vi "opc_client_2.vi"(8 "error in (no error)":errorcluster, 10 "server endpoint URL":string) -> (0 "error out":errorcluster, 1 "Debit":dbl, 2 "Courant":dbl, 4 "Tension":dbl, 5 "temperature":dbl, 6 "Pression":dbl, 7 "etat":string, 11 "OPC UA client refnum out":T1)   [LabVIEW 2019]
uses:
  <vilib>/OPCUA/controls/OPC UA Client Refnum.ctl
  <vilib>/OPCUA/controls/Time Out.ctl
  <vilib>/OPCUA/client/Multiple Read Variant.vi
  <vilib>/OPCUA/NI OPC UA Client.lvlib
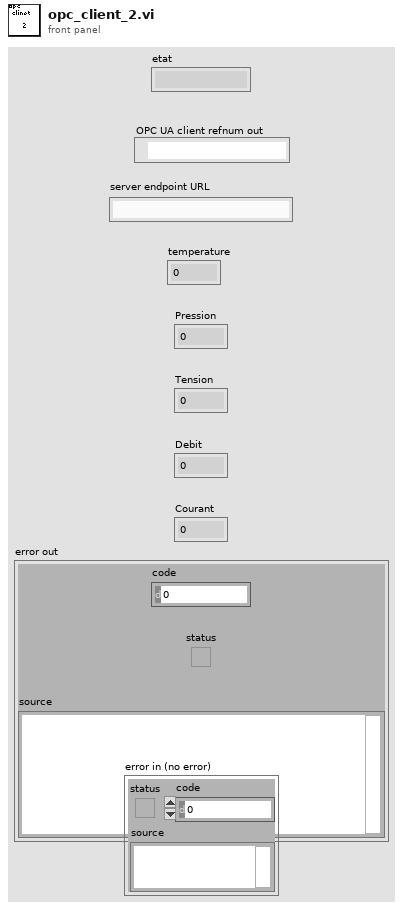
[diagram p1: front panel]
types:
  T1 = typedef "OPC UA Client Refnum.ctl" = refnum<k21>
  T2 = typedef "Time Out.ctl" = u32
  T3 = typedef "Read Variant Result.ctl" = cluster{"node ID":T4, "value ":variant, "timestamp":timestamp, "status":T5}
  T4 = typedef "NodeId.ctl" = string
  T5 = typedef "OPC UA StatusCode.ctl" = u32
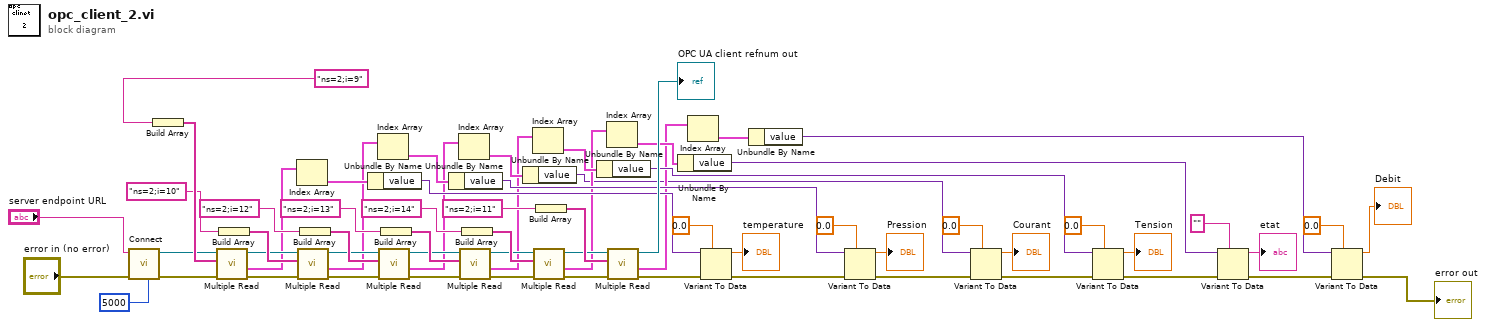
[diagram p0: block diagram]
diagram:
  n1 = call <vilib>:"Connect.vi"("timeout (5000 ms)"=T2 5000, "error in (no error)"="error in (no error)", "server endpoint URL"="server endpoint URL") -> ("error out"=w49:errorcluster, "OPC UA client refnum out"=w63:T1)  [unwired: 6 in, 1 out]
  n2 = Build Array("ns=2;i=9" ("ID")) -> (w64:string[])
  n3 = call-poly <vilib>:"Multiple Read.vi"("error in (no error)"=w49, "node IDs"=w64, "OPC UA client refnum in"=w63) -> ("error out"=w48:errorcluster, "results"=w38:T3[], "OPC UA client refnum out"=w55:T1)  [unwired: 5 in, 1 out]
  n4 = Build Array("ns=2;i=10" ("ID 6")) -> (w56:string[])
  n5 = Index Array(array=w38) -> (element=w37:T3)  [unwired: 1 in]
  n6 = call-poly <vilib>:"Multiple Read.vi"("error in (no error)"=w48, "node IDs"=w56, "OPC UA client refnum in"=w55) -> ("error out"=w47:errorcluster, "results"=w15:T3[], "OPC UA client refnum out"=w54:T1)  [unwired: 5 in, 1 out]
  n7 = Build Array("ns=2;i=12" ("ID 2")) -> (w60:string[])
  n8 = Unbundle By Name(w37) -> ("value"=w35:variant)
  n9 = Index Array(array=w15) -> (element=w19:T3)  [unwired: 1 in]
  n10 = call-poly <vilib>:"Multiple Read.vi"("error in (no error)"=w47, "node IDs"=w60, "OPC UA client refnum in"=w54) -> ("error out"=w46:errorcluster, "results"=w14:T3[], "OPC UA client refnum out"=w53:T1)  [unwired: 5 in, 1 out]
  n11 = Build Array("ns=2;i=13" ("ID 3")) -> (w59:string[])
  n12 = Unbundle By Name(w19) -> ("value"=w17:variant)
  n13 = Index Array(array=w14) -> (element=w30:T3)  [unwired: 1 in]
  n14 = call-poly <vilib>:"Multiple Read.vi"("error in (no error)"=w46, "node IDs"=w59, "OPC UA client refnum in"=w53) -> ("error out"=w45:errorcluster, "results"=w13:T3[], "OPC UA client refnum out"=w52:T1)  [unwired: 5 in, 1 out]
  n15 = Build Array("ns=2;i=14" ("ID 4")) -> (w58:string[])
  n16 = Unbundle By Name(w30) -> ("value"=w2:variant)
  n17 = Index Array(array=w13) -> (element=w27:T3)  [unwired: 1 in]
  n18 = call-poly <vilib>:"Multiple Read.vi"("error in (no error)"=w45, "node IDs"=w58, "OPC UA client refnum in"=w52) -> ("error out"=w44:errorcluster, "results"=w12:T3[], "OPC UA client refnum out"=w51:T1)  [unwired: 5 in, 1 out]
  n19 = Build Array("ns=2;i=11" ("ID 5")) -> (w57:string[])
  n20 = Unbundle By Name(w27) -> ("value"=w25:variant)
  n21 = Index Array(array=w12) -> (element=w33:T3)  [unwired: 1 in]
  n22 = call-poly <vilib>:"Multiple Read.vi"("error in (no error)"=w44, "node IDs"=w57, "OPC UA client refnum in"=w51) -> ("error out"=w4:errorcluster, "results"=w11:T3[], "OPC UA client refnum out"=→"OPC UA client refnum out":T1)  [unwired: 5 in, 1 out]
  n23 = Unbundle By Name(w33) -> ("value"=w32:variant)
  n24 = Index Array(array=w11) -> (element=w23:T3)  [unwired: 1 in]
  n25 = Variant To Data(error in=w4, type=0.0, Variant=w35) -> (data=→"temperature":dbl, error out=w3:errorcluster)
  n26 = Unbundle By Name(w23) -> ("value"=w21:variant)
  n27 = Variant To Data(error in=w3, type=0.0, Variant=w17) -> (data=→"Pression":dbl, error out=w9:errorcluster)
  n28 = Variant To Data(error in=w9, type=0.0, Variant=w2) -> (data=→"Courant":dbl, error out=w8:errorcluster)
  n29 = Variant To Data(error in=w8, type=0.0, Variant=w25) -> (data=→"Tension":dbl, error out=w7:errorcluster)
  n30 = Variant To Data(error in=w7, type="", Variant=w32) -> (data=→"etat":string, error out=w6:errorcluster)
  n31 = Variant To Data(error in=w6, type=0.0, Variant=w21) -> (data=→"Debit":dbl, error out=→"error out":errorcluster)
